vi "4.2.1.vi"() -> ()   [LabVIEW 2018]
panel:
  in  "정지":bool
  out "웨이브폼 차트":dbl(graph)
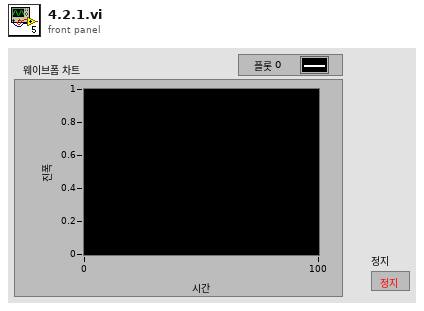
[diagram p1: front panel]
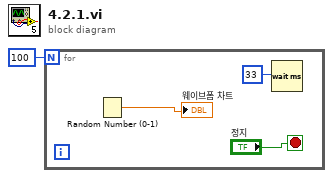
[diagram p0: block diagram]
diagram:
  n1 = for {
    N: 100 -> [_]
    stop <- "정지" stop-if-true
    n2 = Random Number (0-1)() -> (number: 0 to 1=→"웨이브폼 차트":dbl)
    n3 = Wait (ms)(milliseconds to wait=u32 33 ("대기 시간 (ms)")) -> ()  [unwired: 1 out]
  }
